vi "TEST_006.vi"() -> ()   [LabVIEW 2014]
doc: "This example is for the LEGO MINDSTORMS NXT. The program utilizes proportional control to keep an robotic arm at a constant distance above a surface using only a light sensor at the distal end of the arm to measure position."
uses:
  <vilib>/NXT/NXT Controls/ConnectionType.ctl
  <vilib>/NXT/Block Support/NXT_OutputPort.ctl
  <vilib>/NXT/NXTIO Xnodes/NXTIONodeSubVIs/LEGOResetMotors.vi
  <vilib>/NXT/NXTIO Xnodes/NXTIONodeSubVIs/NXTMoveMotors.vi
  <vilib>/NXT/Dual Mode Library/Waits/Wait_Num(msec).vi
  <vilib>/NXT/NXTIO Xnodes/NXTIONodeSubVIs/NXTStopMotors.vi
  <vilib>/NXT/Dual Mode Library/Waits/Wait_Num.vi
  <vilib>/NXT/NXTIO Xnodes/NXTIONodeSubVIs/NXTCheckBattery.vi
  <vilib>/NXT/NXTIO Xnodes/AddressXNode/NXTIOAddress.xnode
  <vilib>/NXT/NXTIO Xnodes/NXTIOXNode/NXTIO.xnode
  <vilib>/NXT/Subs/LVHSConnector.ctl
  <vilib>/NXT/LegoClasses/BrickReference/BrickReference.lvclass
  DLLA.dll
  SensorReader.dll
panel:
  out "전압":sgl
  in  "input t3\n(20~100)":i32
  in  "input t2\n(20~100)":i32
  in  "input w2\n(20~100)":i32
  in  "input w1\n(20~100)":i32
  out "실제 낙하 지점 2":i32
  out "t3 2":dbl
  out "t2 2":dbl
  out "w2 2":dbl
  out "w1 2":dbl
  out "번째":i32
  out "세대":i32
  out "목표 지점":i32
  out "실제 낙하 지점":i32
  out "유전자 정보\n   w1      w2       t2       t3":i32[][](array[numeric])
  in  "0 = 액션 초기화":dbl
  out "t3":dbl
  out "t2":dbl
  out "w2":dbl
  out "w1":dbl
  in  "MODE":dbl
  # "MODE 0 : 기본으로, 학습 및 던지기 작업을 진행합니다.\nMODE 1 : 유전자 정보를 아래 표에 불러옵니다.\nMODE 2 : 사용자가 임의로 입력한 변인에 따라 던집니다."
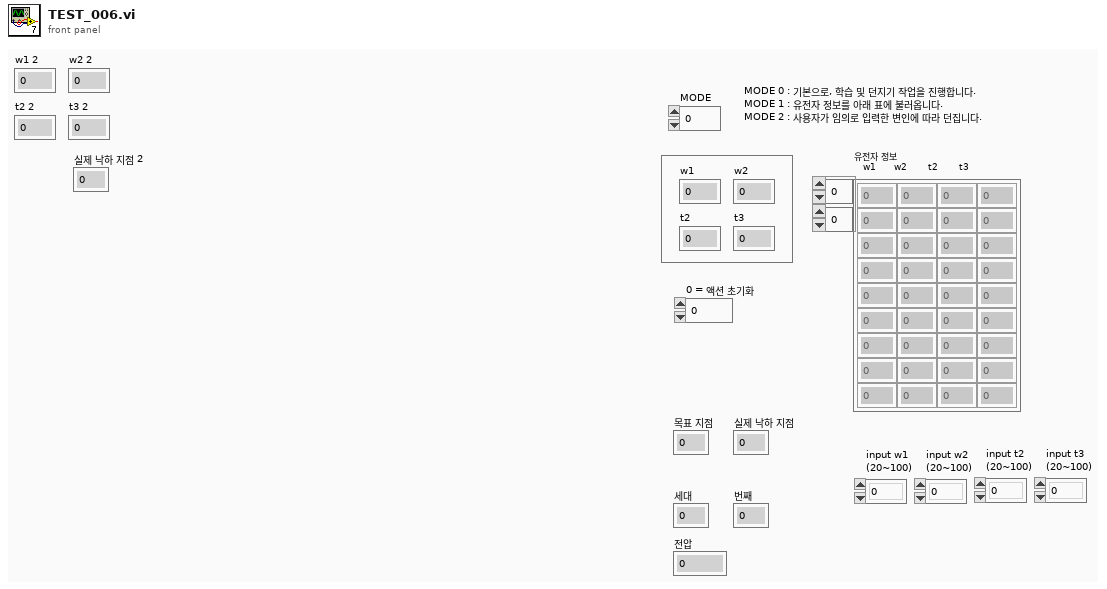
[diagram p1: front panel]
types:
  T1 = typedef "ConnectionType.ctl" = enum16{"Bluetooth", "USB", "WiFi"}
  T2 = typedef "NXT_OutputPort.ctl" = u8
  T3 = cluster{"Output Port":T2, "Output Port 2":T2, "Output Port 3":T2}
  T4 = typedef "LVHSConnector.ctl" = refnum<class "BrickReference.lvclass">
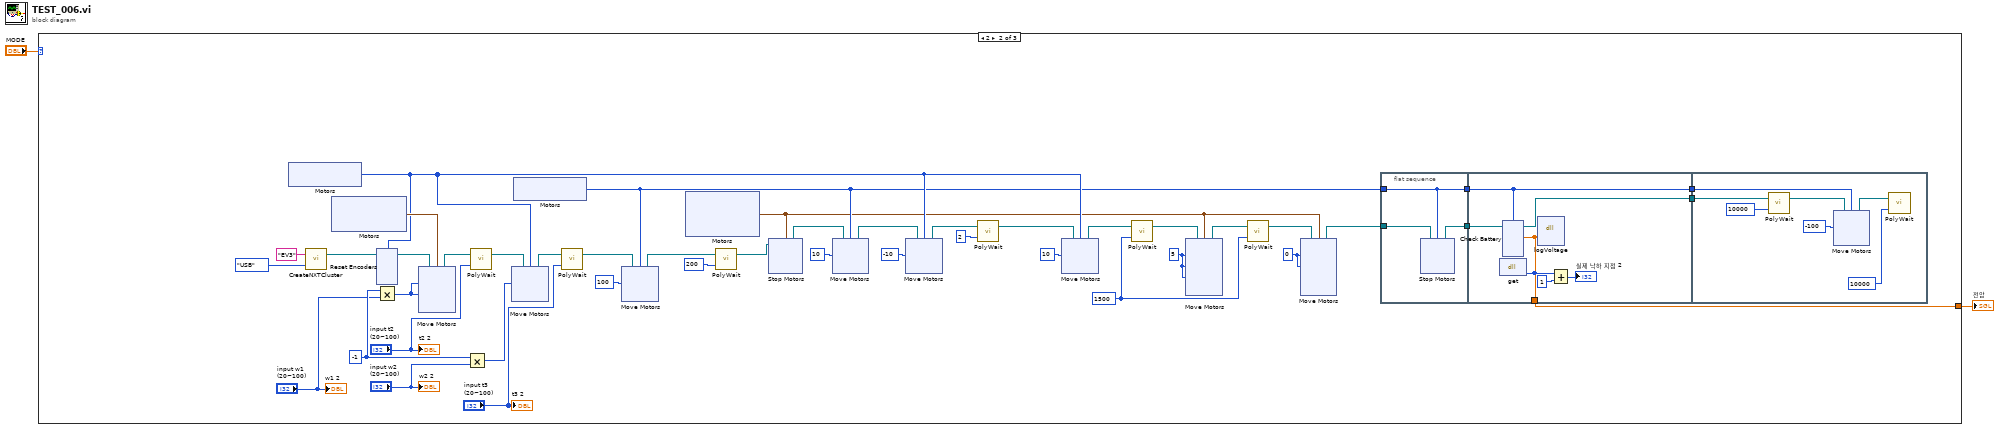
[diagram p0: block diagram]
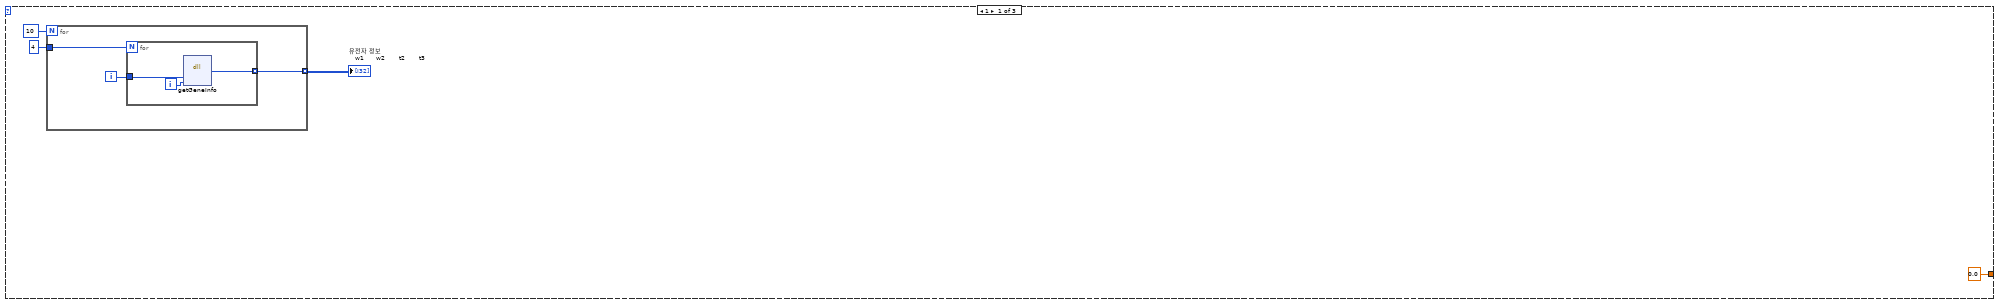
[diagram p2: hidden frame]
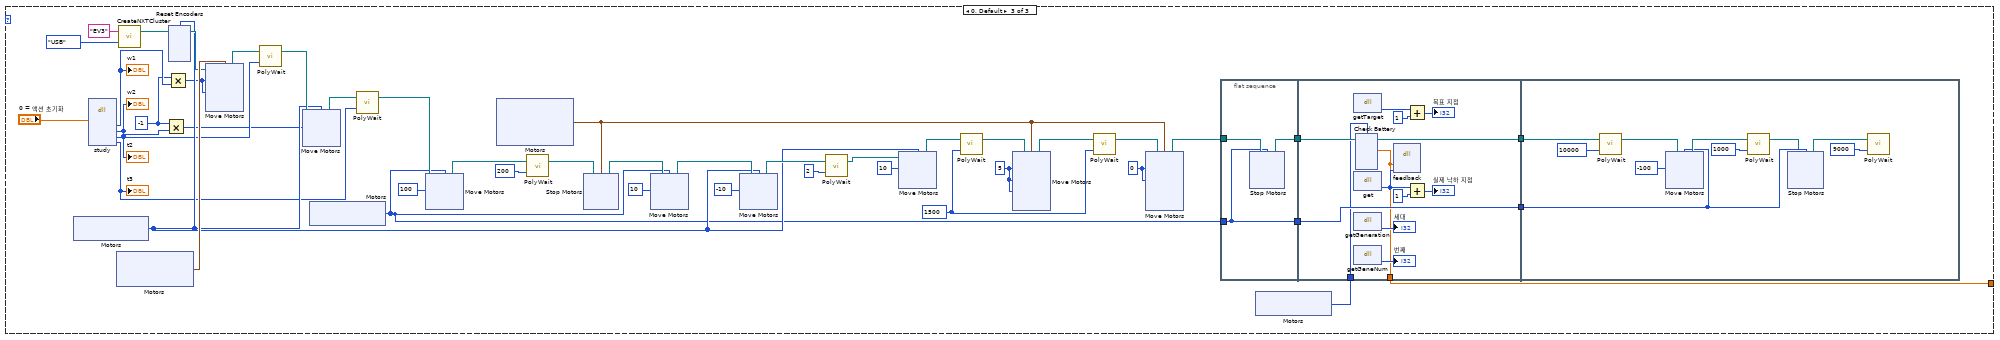
[diagram p3: hidden frame]
diagram:
  n1 = case shown="2" "MODE" {
    tunnel: [sgl 0.0 ("Voltage 1") w13 w166] -> w1
    frame 1 {
      n2 = for {
        N: 10 -> [_]
        tunnel: 4 -> [w9]
        tunnel: [w7] -> w4 mode=indexing
        i -> [w8]
        n3 = for {
          N: w9 -> [_]
          tunnel: w8 -> [w12]
          tunnel: [w10] -> w7 mode=indexing
          i -> [w11]
          n4 = dll-call lib="PTH2dabs CUsers\n컴2실-25DesktopLabVIEW_작업파일-2015-12-28LabVIEW 작업파일DLLA.dll" fn="getGeneInfo"("num"=w12, "attr"=w11) -> ("반환 타입"=w10:i32)  [unwired: 5 in, 2 out]
        }
      }
      "유전자 정보\n   w1      w2       t2       t3" <- w4
    }
    frame 2 {
      w22 = i8 0 ("Power/Speed 1")
      w27 = 5
      w31 = -1
      w23 = 1500
      n5 = xnode "Motors"() -> ("Motor"=w34:T2)
      n6 = call <vilib>:"CreateNXTCluster.vi"("Connection Type"=ConnectionType."USB", "NXT/EV3 name"="EV3") -> ("NXT/EV3"=w18:T4)  [unwired: 2 in]
      n7 = xnode "Motors"() -> ("Motor"=w52:cluster{"Port":T2, "Port":T2})
      n8 = xnode "Reset Encoders"("Motors"=w34, "NXT/EV3"=w18) -> ("NXT/EV3"=w41:T4)
      n9 = Multiply(x=w31, y="input w1\n(20~100)") -> (x*y=w32:i32)
      n10 = xnode "Move Motors"("Power/Speed 2"=w32, "Power/Speed 1"=w32, "Motors"=w52, "NXT/EV3"=w41) -> ("NXT/EV3"=w50:T4)
      n11 = Multiply(x=w31, y="input w2\n(20~100)") -> (x*y=w30:i32)
      n12 = call-poly <vilib>:"PolyWait.vi"("Time (100 msec)"="input t2\n(20~100)", "NXT/EV3"=w50) -> ("NXT/EV3"=w49:T4)  [unwired: 2 in]
      n13 = xnode "Move Motors"("Power/Speed 1"=w30, "Motors"=w34, "NXT/EV3"=w49) -> ("NXT/EV3"=w48:T4)
      n14 = xnode "Motors"() -> ("Motor"=w29:T2)
      n15 = call-poly <vilib>:"PolyWait.vi"("Time (100 msec)"="input t3\n(20~100)", "NXT/EV3"=w48) -> ("NXT/EV3"=w47:T4)  [unwired: 2 in]
      n16 = xnode "Move Motors"("Power/Speed 1"=100, "Motors"=w29, "NXT/EV3"=w47) -> ("NXT/EV3"=w46:T4)
      n17 = xnode "Motors"() -> ("Motor"=w26:cluster{"Port":T2, "Port":T2, "Port":T2})
      n18 = call-poly <vilib>:"PolyWait.vi"("Time (100 msec)"=200, "NXT/EV3"=w46) -> ("NXT/EV3"=w43:T4)  [unwired: 2 in]
      n19 = xnode "Stop Motors"("Motors"=w26, "NXT/EV3"=w43) -> ("NXT/EV3"=w40:T4)
      n20 = xnode "Move Motors"("Power/Speed 1"=10, "Motors"=w29, "NXT/EV3"=w40) -> ("NXT/EV3"=w38:T4)
      n21 = xnode "Move Motors"("Power/Speed 1"=-10, "Motors"=w34, "NXT/EV3"=w38) -> ("NXT/EV3"=w37:T4)
      n22 = call-poly <vilib>:"PolyWait.vi"("Time (1 sec)"=2, "NXT/EV3"=w37) -> ("NXT/EV3"=w36:T4)  [unwired: 2 in]
      n23 = xnode "Move Motors"("Power/Speed 1"=10, "Motors"=w34, "NXT/EV3"=w36) -> ("NXT/EV3"=w35:T4)
      n24 = call-poly <vilib>:"PolyWait.vi"("Time (100 msec)"=w23, "NXT/EV3"=w35) -> ("NXT/EV3"=w28:T4)  [unwired: 2 in]
      n25 = xnode "Move Motors"("Power/Speed 3"=w27, "Power/Speed 2"=w27, "Power/Speed 1"=w27, "Motors"=w26, "NXT/EV3"=w28) -> ("NXT/EV3"=w25:T4)
      n26 = call-poly <vilib>:"PolyWait.vi"("Time (100 msec)"=w23, "NXT/EV3"=w25) -> ("NXT/EV3"=w24:T4)  [unwired: 2 in]
      n27 = xnode "Move Motors"("Power/Speed 2"=w22, "Power/Speed 1"=w22, "Motors"=w26, "NXT/EV3"=w24) -> ("NXT/EV3"=w21:T4)  [unwired: 1 in]
      n28 = flat-sequence {
        tunnel: w29 -> [w57]
        tunnel: w21 -> [w58]
        tunnel: [w59] -> w56
        tunnel: [w57] -> w55
        tunnel: w56 -> [w70]
        tunnel: [w69] -> w54
        tunnel: [w68] -> w53
        tunnel: w55 -> [w68]
        tunnel: [w66] -> w13
        tunnel: w54 -> [w83]
        tunnel: w53 -> [w78]
        frame #0 {
          n29 = xnode "Stop Motors"("Motors"=w57, "NXT/EV3"=w58) -> ("NXT/EV3"=w59:T4)
        }
        frame #1 {
          n30 = dll-call lib="PTH2labs CUsers\n컴2실-25DesktopLabVIEW_작업파일-2015-12-28LabVIEW 작업파일SensorReader.dll" fn="get"() -> ("반환 타입"=w65:i32)  [unwired: 3 in, 2 out]
          n31 = xnode "Check Battery"("Motors"=w68, "NXT/EV3"=w70) -> ("Voltage 1"=w66:sgl, "NXT/EV3"=w69:T4)
          n32 = dll-call lib="PTH2dabs CUsers\n컴2실-25DesktopLabVIEW_작업파일-2015-12-28LabVIEW 작업파일DLLA.dll" fn="logVoltage"("voltage"=w66, "value"=w65) -> ()  [unwired: 6 in, 2 out]
          n33 = Add(x=w65, y=1) -> (x+y=→"실제 낙하 지점 2":i32)
        }
        frame #2 {
          n34 = call-poly <vilib>:"PolyWait.vi"("Time (100 msec)"=10000, "NXT/EV3"=w83) -> ("NXT/EV3"=w77:T4)  [unwired: 2 in]
          n35 = xnode "Move Motors"("Power/Speed 1"=-100, "Motors"=w78, "NXT/EV3"=w77) -> ("NXT/EV3"=w80:T4)
          n36 = call-poly <vilib>:"PolyWait.vi"("Time (100 msec)"=u32 10000, "NXT/EV3"=w80) -> ()  [unwired: 2 in, 1 out]
        }
      }
      "w1 2" <- "input w1\n(20~100)"
      "w2 2" <- "input w2\n(20~100)"
      "t2 2" <- "input t2\n(20~100)"
      "t3 2" <- "input t3\n(20~100)"
    }
    frame 0, Default {
      w175 = i8 0 ("Power/Speed 1")
      w180 = 5
      w185 = -1
      w176 = 1500
      n37 = xnode "Motors"() -> ("Motor"=w192:T2)
      n38 = dll-call lib="PTH2dabs CUsers\n컴2실-25DesktopLabVIEW_작업파일-2015-12-28LabVIEW 작업파일DLLA.dll" fn="study"("state"="0 = 액션 초기화") -> ("w1"=w187:i32, "w2"=w186:i32, "t2"=w190:i32, "t3"=w189:i32)  [unwired: 9 in, 2 out]
      "w1" <- w187
      "w2" <- w186
      "t2" <- w190
      "t3" <- w189
      n39 = xnode "Motors"() -> ("Motor"=w210:cluster{"Port":T2, "Port":T2})
      n40 = call <vilib>:"CreateNXTCluster.vi"("Connection Type"=ConnectionType."USB", "NXT/EV3 name"="EV3") -> ("NXT/EV3"=w171:T4)  [unwired: 2 in]
      n41 = Multiply(x=w185, y=w186) -> (x*y=w184:i32)
      n42 = Multiply(x=w185, y=w187) -> (x*y=w188:i32)
      n43 = xnode "Reset Encoders"("Motors"=w192, "NXT/EV3"=w171) -> ("NXT/EV3"=w199:T4)
      n44 = xnode "Move Motors"("Power/Speed 2"=w188, "Power/Speed 1"=w188, "Motors"=w210, "NXT/EV3"=w199) -> ("NXT/EV3"=w208:T4)
      n45 = call-poly <vilib>:"PolyWait.vi"("Time (100 msec)"=w190, "NXT/EV3"=w208) -> ("NXT/EV3"=w207:T4)  [unwired: 2 in]
      n46 = xnode "Move Motors"("Power/Speed 1"=w184, "Motors"=w192, "NXT/EV3"=w207) -> ("NXT/EV3"=w206:T4)
      n47 = xnode "Motors"() -> ("Motor"=w182:T2)
      n48 = call-poly <vilib>:"PolyWait.vi"("Time (100 msec)"=w189, "NXT/EV3"=w206) -> ("NXT/EV3"=w205:T4)  [unwired: 2 in]
      n49 = xnode "Move Motors"("Power/Speed 1"=100, "Motors"=w182, "NXT/EV3"=w205) -> ("NXT/EV3"=w204:T4)
      n50 = xnode "Motors"() -> ("Motor"=w179:cluster{"Port":T2, "Port":T2, "Port":T2})
      n51 = call-poly <vilib>:"PolyWait.vi"("Time (100 msec)"=200, "NXT/EV3"=w204) -> ("NXT/EV3"=w201:T4)  [unwired: 2 in]
      n52 = xnode "Stop Motors"("Motors"=w179, "NXT/EV3"=w201) -> ("NXT/EV3"=w198:T4)
      n53 = xnode "Move Motors"("Power/Speed 1"=10, "Motors"=w182, "NXT/EV3"=w198) -> ("NXT/EV3"=w196:T4)
      n54 = xnode "Move Motors"("Power/Speed 1"=-10, "Motors"=w192, "NXT/EV3"=w196) -> ("NXT/EV3"=w195:T4)
      n55 = call-poly <vilib>:"PolyWait.vi"("Time (1 sec)"=2, "NXT/EV3"=w195) -> ("NXT/EV3"=w194:T4)  [unwired: 2 in]
      n56 = xnode "Move Motors"("Power/Speed 1"=10, "Motors"=w192, "NXT/EV3"=w194) -> ("NXT/EV3"=w193:T4)
      n57 = call-poly <vilib>:"PolyWait.vi"("Time (100 msec)"=w176, "NXT/EV3"=w193) -> ("NXT/EV3"=w181:T4)  [unwired: 2 in]
      n58 = xnode "Move Motors"("Power/Speed 3"=w180, "Power/Speed 2"=w180, "Power/Speed 1"=w180, "Motors"=w179, "NXT/EV3"=w181) -> ("NXT/EV3"=w178:T4)
      n59 = call-poly <vilib>:"PolyWait.vi"("Time (100 msec)"=w176, "NXT/EV3"=w178) -> ("NXT/EV3"=w177:T4)  [unwired: 2 in]
      n60 = xnode "Move Motors"("Power/Speed 2"=w175, "Power/Speed 1"=w175, "Motors"=w179, "NXT/EV3"=w177) -> ("NXT/EV3"=w174:T4)  [unwired: 1 in]
      n61 = flat-sequence {
        tunnel: w182 -> [w212]
        tunnel: w174 -> [w213]
        tunnel: [w214] -> w170
        tunnel: [w212] -> w167
        tunnel: w170 -> [w224]
        tunnel: [w223] -> w169
        tunnel: [w222] -> w168
        tunnel: w167 -> [w222]
        tunnel: [w221] -> w166
        tunnel: w165 -> [w220]
        tunnel: w169 -> [w247]
        tunnel: w168 -> [w240]
        frame #0 {
          n62 = xnode "Stop Motors"("Motors"=w212, "NXT/EV3"=w213) -> ("NXT/EV3"=w214:T4)
        }
        frame #1 {
          n63 = dll-call lib="PTH2dabs CUsers\n컴2실-25DesktopLabVIEW_작업파일-2015-12-28LabVIEW 작업파일DLLA.dll" fn="getTarget"() -> ("반환 타입"=w228:i32)  [unwired: 3 in, 2 out]
          n64 = dll-call lib="PTH2labs CUsers\n컴2실-25DesktopLabVIEW_작업파일-2015-12-28LabVIEW 작업파일SensorReader.dll" fn="get"() -> ("반환 타입"=w231:i32)  [unwired: 3 in, 2 out]
          n65 = dll-call lib="PTH2dabs CUsers\n컴2실-25DesktopLabVIEW_작업파일-2015-12-28LabVIEW 작업파일DLLA.dll" fn="getGeneration"() -> ("반환 타입"=→"세대":i32)  [unwired: 3 in, 2 out]
          n66 = dll-call lib="PTH2dabs CUsers\n컴2실-25DesktopLabVIEW_작업파일-2015-12-28LabVIEW 작업파일DLLA.dll" fn="getGeneNum"() -> ("반환 타입"=→"번째":i32)  [unwired: 3 in, 2 out]
          n67 = xnode "Check Battery"("Motors"=w220, "NXT/EV3"=w224) -> ("Voltage 1"=w221:sgl, "NXT/EV3"=w223:T4)
          n68 = dll-call lib="PTH2dabs CUsers\n컴2실-25DesktopLabVIEW_작업파일-2015-12-28LabVIEW 작업파일DLLA.dll" fn="feedback"("voltage"=w221, "value"=w231) -> ()  [unwired: 6 in, 2 out]
          n69 = Add(x=w228, y=1) -> (x+y=→"목표 지점":i32)
          n70 = Add(x=w231, y=1) -> (x+y=→"실제 낙하 지점":i32)
        }
        frame #2 {
          n71 = call-poly <vilib>:"PolyWait.vi"("Time (100 msec)"=10000, "NXT/EV3"=w247) -> ("NXT/EV3"=w242:T4)  [unwired: 2 in]
          n72 = xnode "Move Motors"("Power/Speed 1"=-100, "Motors"=w240, "NXT/EV3"=w242) -> ("NXT/EV3"=w244:T4)
          n73 = call-poly <vilib>:"PolyWait.vi"("Time (100 msec)"=u32 1000, "NXT/EV3"=w244) -> ("NXT/EV3"=w239:T4)  [unwired: 2 in]
          n74 = xnode "Stop Motors"("Motors"=w240, "NXT/EV3"=w239) -> ("NXT/EV3"=w238:T4)
          n75 = call-poly <vilib>:"PolyWait.vi"("Time (100 msec)"=u32 9000, "NXT/EV3"=w238) -> ()  [unwired: 2 in, 1 out]
        }
      }
      n76 = xnode "Motors"() -> ("Motor"=w165:T2)
    }
  }
  "전압" <- w1
